vi "nivsfpga_AddTemplateToProject.vi"(8 "error in (no error)":errorcluster, 11 "FPGA Target ref in":refnum<vi>) -> (0 "error out":errorcluster, 1 "VI Project Item Reference":refnum<vi>, 3 "FPGA Target ref out":refnum<vi>)   [LabVIEW 2018]
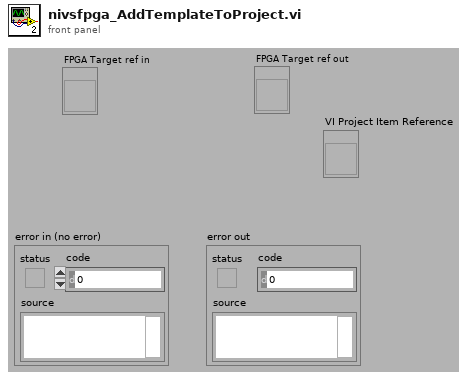
[diagram p1: front panel]
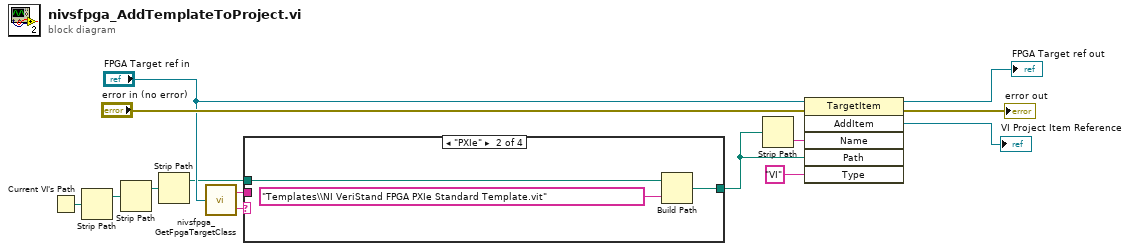
[diagram p0: block diagram]
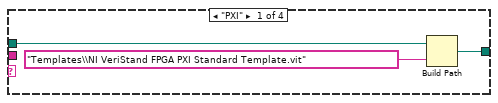
[diagram p2: hidden frame]
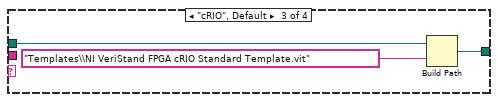
[diagram p3: hidden frame]
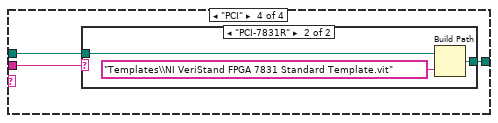
[diagram p4: hidden frame]
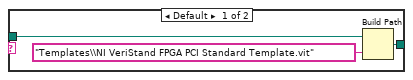
[diagram p5: hidden frame]
diagram:
  n1 = Current VI's Path() -> (path=w2:path)
  n2 = Strip Path(path=w2) -> (stripped path=w3:path)  [unwired: 1 out]
  n3 = Strip Path(path=w3) -> (stripped path=w11:path)  [unwired: 1 out]
  n4 = Strip Path(path=w11) -> (stripped path=w4:path)  [unwired: 1 out]
  n5 = call <userlib>:"nivsfpga_GetFpgaTargetClass.vi"("FPGA target"="FPGA Target ref in") -> ("Target"=w1:string, "Platform"=w12:string)
  n6 = case shown="\"PXIe\"" w12 {
    tunnel: w4 -> [w16 w19 w23 w25]
    tunnel: [w15 w18 w22 w24] -> w10
    tunnel: w1 -> [_ _ _ w26]
    frame "PXI" {
      n7 = Build Path(base path=w16, name or relative path="Templates\\NI VeriStand FPGA PXI Standard Template.vit") -> (appended path=w15:path)
    }
    frame "PXIe" {
      n8 = Build Path(base path=w19, name or relative path="Templates\\NI VeriStand FPGA PXIe Standard Template.vit") -> (appended path=w18:path)
    }
    frame "cRIO", Default {
      n9 = Build Path(base path=w23, name or relative path="Templates\\NI VeriStand FPGA cRIO Standard Template.vit") -> (appended path=w22:path)
    }
    frame "PCI" {
      n10 = case shown="\"PCI-7831R\"" w26 {
        tunnel: w25 -> [w28 w31]
        tunnel: [w27 w30] -> w24
        frame Default {
          n11 = Build Path(base path=w28, name or relative path="Templates\\NI VeriStand FPGA PCI Standard Template.vit") -> (appended path=w27:path)
        }
        frame "PCI-7831R" {
          n12 = Build Path(base path=w31, name or relative path="Templates\\NI VeriStand FPGA 7831 Standard Template.vit") -> (appended path=w30:path)
        }
      }
    }
  }
  n13 = Strip Path(path=w10) -> (name=w7:string)  [unwired: 1 out]
  n14 = invoke class="TargetItem" method="AddItem"(reference="FPGA Target ref in", error in="error in (no error)", "Name"=w7, "Path"=w10, "Type"="VI") -> (reference out=→"FPGA Target ref out":refnum<vi>, error out=→"error out":errorcluster, "AddItem"=→"VI Project Item Reference":refnum<vi>)  [unwired: 1 in, 3 out]
